vi "Remove-inactive-client.vi"(8 "error in (no error)":errorcluster, 10 "Client index":i32, 11 "ModComm in":T1) -> (0 "error out":errorcluster, 3 "ModComm out":T1)   [LabVIEW 2013, in "Server.lvlib" / "Server.lvclass"]
uses:
  Server.lvclass
  Object-reference.ctl
  UI-messages.ctl
  Server.lvclass/Server.ctl
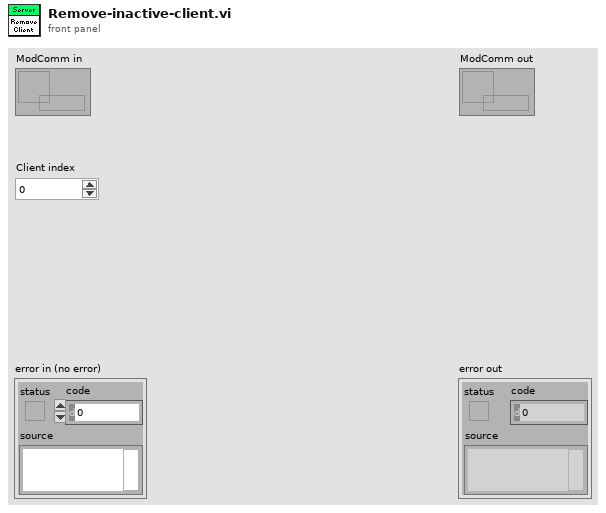
[diagram p1: front panel]
types:
  T1 = typedef "Server.lvlib/Server.lvclass/Object-reference.ctl" = refnum<data-value>
  T2 = typedef "Server.lvlib/Server.lvclass/UI-messages.ctl" = enum16{"Time out", "User cancel", "Module cancel", "Client inactivity", "Client limit", "Client started"}
  T3 = typedef "Server.lvlib/Server.lvclass/Supported-module-types.ctl" = enum16{"Server", "All", "BeamControl", "PowderDeposition", "StrategyParser", "CameraVision", "MaterialCharacterization", "StatusMonitor", "SLMSimulation", "LaserCharacterization"}
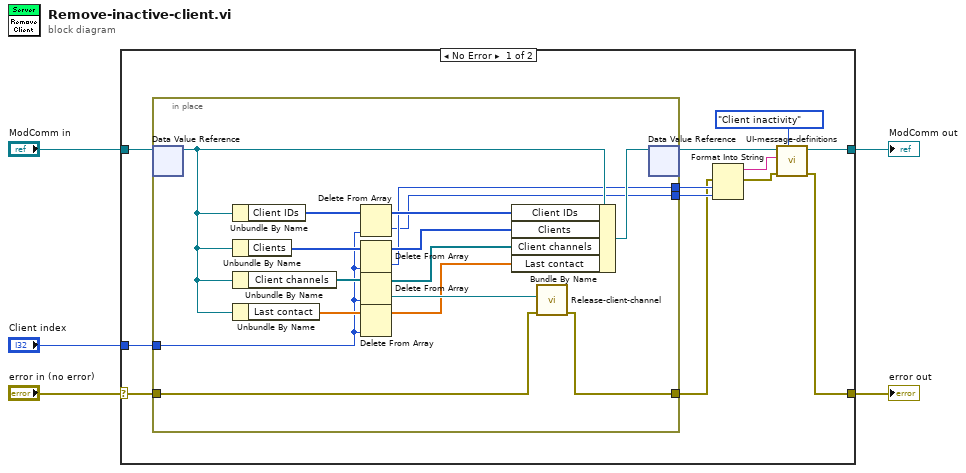
[diagram p0: block diagram]
diagram:
  n1 = case shown="No Error" "error in (no error)" {
    selector: "error in (no error)" -> [w15 w35]
    tunnel: [w12 w35] -> w4
    tunnel: [w13 w34] -> w2
    tunnel: "ModComm in" -> [w17 w34]
    tunnel: "Client index" -> [w16 _]
    frame No Error {
      n2 = in-place {
        in-place-border: w16 -> [w29]
        in-place-border: w15 -> [w27]
        in-place-border: [w20] -> w8
        in-place-border: [w19] -> w11
        in-place-border: [w18] -> w10
        n3 = in-place-dvr #1(w17) -> (w21:refnum<class "Server.lvclass">)  [unwired: 1 out]
        n4 = Unbundle By Name(w21) -> ("Client IDs"=w33:i32[])
        n5 = Unbundle By Name(w21) -> ("Clients"=w32:T3[])
        n6 = Unbundle By Name(w21) -> ("Client channels"=w31:refnum<queue>[])
        n7 = Unbundle By Name(w21) -> ("Last contact"=w30:dbl[])
        n8 = Delete From Array(array=w33, index=w29) -> (deleted portion=w18:i32, array with subset deleted=w26:i32[])  [unwired: 1 in]
        n9 = Delete From Array(array=w32, index=w29) -> (deleted portion=w19:T3, array with subset deleted=w25:T3[])  [unwired: 1 in]
        n10 = Delete From Array(array=w31, index=w29) -> (deleted portion=w28:refnum<queue>, array with subset deleted=w24:refnum<queue>[])  [unwired: 1 in]
        n11 = Delete From Array(array=w30, index=w29) -> (array with subset deleted=w23:dbl[])  [unwired: 1 in, 1 out]
        n12 = Bundle By Name(cluster=w21, "Client IDs"=w26, "Clients"=w25, "Client channels"=w24, "Last contact"=w23) -> (w22:refnum<class "Server.lvclass">)
        n13 = call "Release-client-channel.vi"("error in (no error)"=w27, "Comm channel"=w28) -> ("error out"=w20:errorcluster)  [unwired: 9 in]
        n14 = in-place-dvr #1(w22) -> (w14:T1)  [unwired: 1 out]
      }
      n15 = Format Into String(error in=w8, w11, w10) -> (resulting string=w6:string, error out=w9:errorcluster)  [unwired: 2 in]
      n16 = call "UI-message-definitions.vi"("Message"=UI-messages."Client inactivity", "error in (no error)"=w9, "Additional text"=w6, "ModComm in"=w14) -> ("error out"=w12:errorcluster, "ModComm out"=w13:T1)  [unwired: 6 in]
    }
    frame Error {
    }
  }
  "error out" <- w4
  "ModComm out" <- w2
